vi "Lakeshore_init.vi"(8 "error in (no error)":errorcluster, 11 "VISA In":refnum<visa-resource-name>) -> (0 "error out":errorcluster, 1 "Init Status":bool)   [LabVIEW 2018]
uses:
  <vilib>/Instr/_visa.llb/VISA Open Access Mode.ctl
  <vilib>/Instr/_visa.llb/VISA Flush IO Buffer Mask.ctl
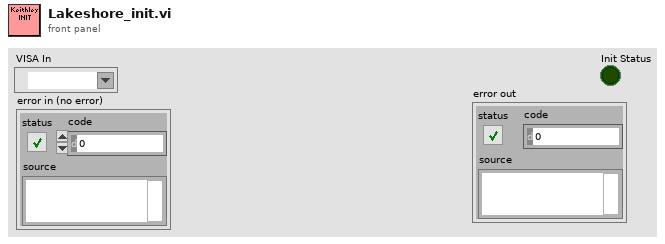
[diagram p1: front panel]
types:
  T1 = typedef "VISA Flush IO Buffer Mask.ctl" = u16
  T2 = typedef "VISA Open Access Mode.ctl" = u32
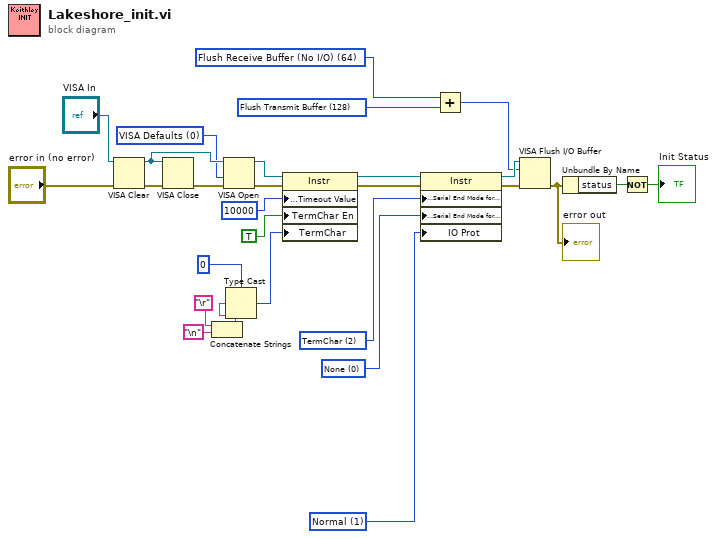
[diagram p0: block diagram]
diagram:
  w9 = T1 128 items=["Flush Receive Buffer"=16, "Write Transmit Buffer to Device"=32, "Flush Receive Buffer (No I/O)"=64, "Flush Transmit Buffer"=128] ("Mask")
  w10 = T1 64 items=["Flush Receive Buffer"=16, "Write Transmit Buffer to Device"=32, "Flush Receive Buffer (No I/O)"=64, "Flush Transmit Buffer"=128] ("Mask")
  w15 = u16 2 items=["None", "LastBit", "TermChar"] ("Serial Settings:Serial End Mode for Reads")
  w1 = u16 1 items=["Normal"=1, "VXI/FDC"=2, "GPIB/HS488"=3, "Serial-TCPIP-USB/488 Strings"=4, "USBTMC/Vendor-Specific"=5] ("Message Based Settings:IO Protocol")
  w16 = u16 0 items=["None", "LastBit", "TermChar"] ("Serial Settings:Serial End Mode for Reads")
  w23 = T2 0 items=["VISA Defaults"=0, "Exclusive Lock"=1, "Load Configured Settings"=4] ("Access Mode")
  n1 = VISA Clear(VISA resource name="VISA In", error in (no error)="error in (no error)") -> (VISA resource name out=w24:refnum<visa-resource-name>, error out=w28:errorcluster)
  n2 = VISA Close(VISA resource name=w24, error in (no error)=w28) -> (error out=w25:errorcluster)
  n3 = Concatenate Strings("\r", "\n") -> (w2:string)
  n4 = VISA Open(access mode=w23, error in (no error)=w25, VISA resource name=w24) -> (VISA resource name=w19:refnum<visa-resource-name>, error out=w18:errorcluster)  [unwired: 2 out]
  n5 = Type Cast(type=u8 0 ("Message Based Settings:Termination Character"), x=w2) -> (*(type *) &x=w20:u8)
  n6 = property on="Property Node" class="Instr"(reference=w19, error in=w18, "General Settings:Timeout Value"=u32 10000, "TermChar En"=TRUE ("Message Based Settings:Termination Character Enable"), "TermChar"=w20) -> (reference out=w14:refnum<visa-resource-name>, error out=w13:errorcluster)
  n7 = property on="Property Node" class="Instr"(reference=w14, error in=w13, "Serial Settings:Serial End Mode for Reads"=w15, "Serial Settings:Serial End Mode for Writes"=w16, "IO Prot"=w1) -> (reference out=w11:refnum<visa-resource-name>, error out=w12:errorcluster)
  n8 = Add(x=w10, y=w9) -> (x+y=w8:T1)
  n9 = VISA Flush I/O Buffer(VISA resource name=w11, mask (16)=w8, error in (no error)=w12) -> (error out=w6:errorcluster)  [unwired: 1 out]
  "error out" <- w6
  n10 = Unbundle By Name(w6) -> ("status"=w5:bool)
  n11 = Not(x=w5) -> (.not. x?=→"Init Status":bool)
